vi "DAQ AI one shot ch 2 3.vi"(0 "device name":tag="Dev1", 1 "timeout (s)":dbl=1.0 format="%0.2f", 2 "stop (T)":bool=TRUE, 11 "error in":errorcluster, 12 "physical channels":string[](array[string])=["ai2", "ai3"], 13 "channel names":string[](array[string])=["Thermistor", "Heater"]) -> (4 "device name out":tag="Dev1", 6 "thermistor voltage":dbl, 10 "heater voltage":dbl, 14 "data":dynamicdata(waveform) caption="dynamic data", 15 "error out":errorcluster)   [LabVIEW 2019]
doc: "NI ELVIS \nAsynchronous AI one shot \nchannels 2 3 \nbug thermistor and heater\n\ncreated with DAQmx assistant\n\nPaul K Dixon\nP3600\nCSUSB Physics\n\n\nCreates, edits, and runs tasks using NI-DAQmx. Refer to the NI-DAQmx Readme for a complete listing of devices NI-DAQmx supports.\n\nWhen you place this Express VI on the block diagram, the DAQ Assistant launches to create a new task. After you create a task, you can double-click the DAQ Assistant Express VI to edit that task. For continuous measurement or generation, place a while loop around the DAQ Assistant Express VI."
uses:
  <vilib>/DAQmx/read.llb/DAQmx Read.vi
  <vilib>/DAQmx/read.llb/DAQmx Read (Analog 1D DBL NChan 1Samp).vi
  <vilib>/DAQmx/create/channels.llb/DAQmx Create Channel (TEDS-AI-Voltage-Basic).vi
  <vilib>/DAQmx/create/channels.llb/DAQmx Create Channel (AI-Voltage-Basic).vi
  <vilib>/DAQmx/miscellaneous.llb/DAQmx Fill In Error Info.vi
panel:
  # "DAQmx NI ELVIS \nAsynchronous AI one shot \nchannels 2 3  \nbug thermistor and heater"
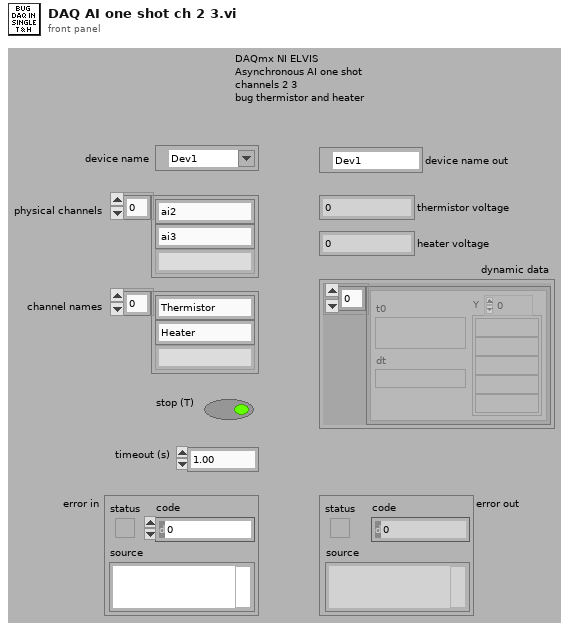
[diagram p1: front panel]
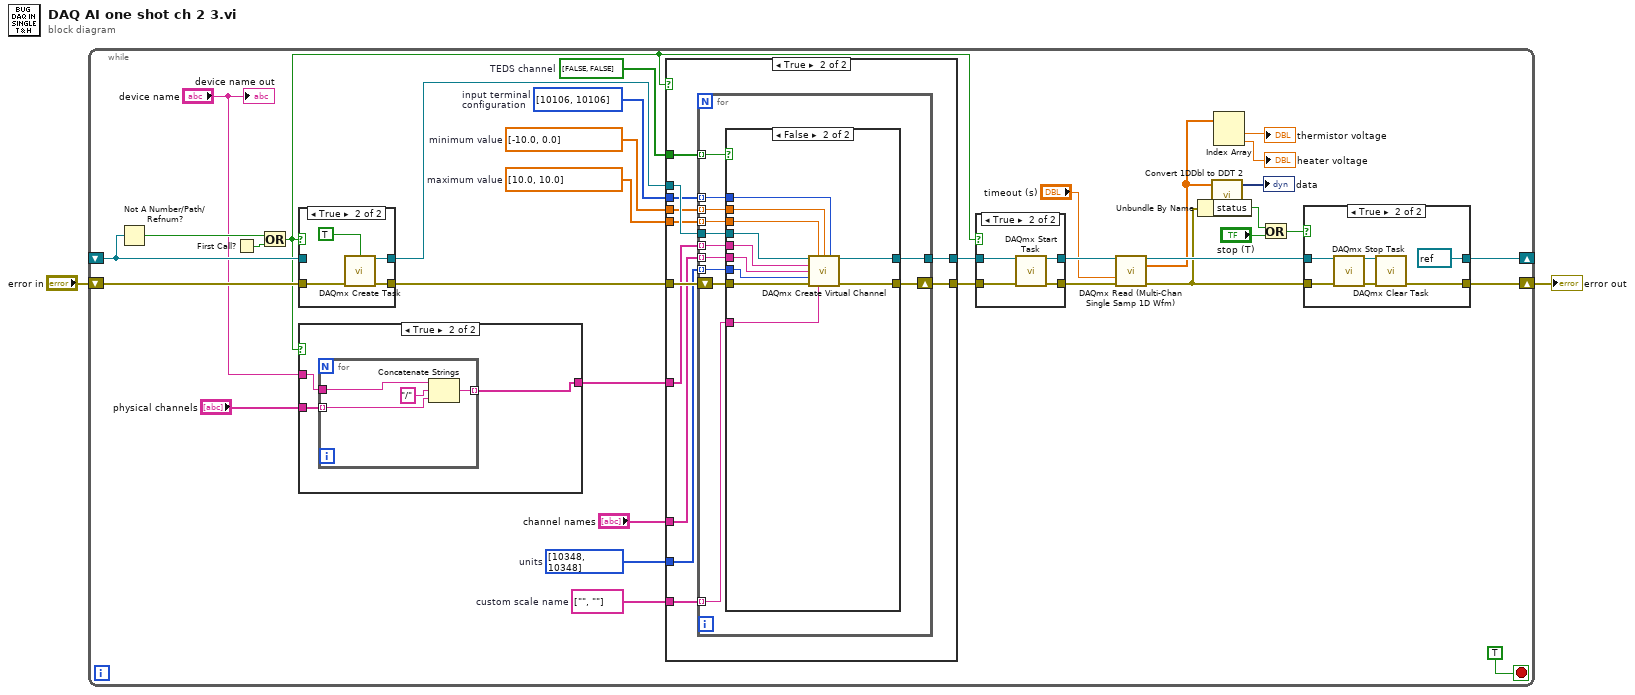
[diagram p0: block diagram]
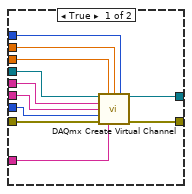
[diagram p5: hidden frame]
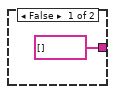
[diagram p6: hidden frame]
diagram:
  n1 = while {
    shift-right: [w12] -> _
    shift-left: _ -> [w33]
    shift-right: [w10] -> w1
    shift-left: "error in" -> [w34]
    stop <- TRUE stop-if-true
    w20 = bool[] [FALSE, FALSE]  # TEDS channel
    w21 = string[] ["", ""]  # custom scale name
    w22 = i32[] [10348, 10348] items=["Volts"=10348, "From TEDS"=12516, "From Custom Scale"=10065]  # units
    w25 = dbl[] [10.0, 10.0]  # maximum value
    w26 = dbl[] [-10.0, 0.0]  # minimum value
    w27 = i32[] [10106, 10106] items=["default"=-1, "RSE"=10083, "NRSE"=10078, "Differential"=10106, "Pseudodifferential"=12529]  # input terminal configuration
    n2 = Not A Number/Path/Refnum?(number/path/refnum=w33) -> (NaN/Path/Refnum?=w32:bool)
    n3 = First Call?() -> (First Call?: T/F=w35:bool)
    n4 = Or(x=w32, y=w35) -> (x .or. y?=w19:bool)
    n5 = case shown="True" w19 {
      tunnel: [w108 w112] -> w29
      tunnel: w33 -> [w108 _]
      tunnel: [w107 w111] -> w28
      tunnel: w34 -> [w107 w109]
      frame False {
      }
      frame True {
        n6 = call <vilib>:"DAQmx Create Task.vi"("auto cleanup"=TRUE, "error in"=w109) -> ("task out"=w112:refnum<k21>, "error out"=w111:errorcluster)  [unwired: 12 in]
      }
    }
    n7 = case shown="True" w19 {
      tunnel: [string[] [] w102] -> w24
      tunnel: "device name" -> [_ w101]
      tunnel: "physical channels" -> [_ w100]
      frame False {
      }
      frame True {
        n8 = for {
          tunnel: [w106] -> w102 mode=indexing
          tunnel: w101 -> [w105]
          tunnel: w100 -> [w103] mode=indexing
          n9 = Concatenate Strings(w105, "/" ("string"), w103) -> (w106:string)
        }
      }
    }
    n10 = case shown="True" w19 {
      tunnel: [w52 w62] -> w18
      tunnel: w29 -> [w52 w64]
      tunnel: [w51 w61] -> w17
      tunnel: w28 -> [w51 w63]
      tunnel: w27 -> [_ w60]
      tunnel: w26 -> [_ w59]
      tunnel: w25 -> [_ w58]
      tunnel: w24 -> [_ w57]
      tunnel: "channel names" -> [_ w56]
      tunnel: w22 -> [_ w55]
      tunnel: w21 -> [_ w54]
      tunnel: w20 -> [_ w53]
      frame False {
      }
      frame True {
        n11 = for {
          tunnel: w64 -> [w76]
          tunnel: [w74] -> w62
          tunnel: w60 -> [w72] mode=indexing
          tunnel: w59 -> [w71] mode=indexing
          tunnel: w58 -> [w70] mode=indexing
          tunnel: w57 -> [w69] mode=indexing
          tunnel: w56 -> [w68] mode=indexing
          tunnel: w55 -> [w67] mode=indexing
          tunnel: w54 -> [w66] mode=indexing
          shift-right: [w73] -> w61
          shift-left: w63 -> [w75]
          tunnel: w53 -> [w65] mode=indexing
          n12 = case shown="False" w65 {
            tunnel: w76 -> [w87 w98]
            tunnel: w75 -> [w86 w97]
            tunnel: [w85 w96] -> w74
            tunnel: [w84 w95] -> w73
            tunnel: w72 -> [w83 w94]
            tunnel: w71 -> [w82 w93]
            tunnel: w70 -> [w81 w92]
            tunnel: w69 -> [w80 w91]
            tunnel: w68 -> [w79 w90]
            tunnel: w67 -> [w78 w89]
            tunnel: w66 -> [w77 w88]
            frame True {
              n13 = call-poly <vilib>:"DAQmx Create Virtual Channel.vi"("task in"=w87, "maximum value"=w81, "minimum value"=w82, "input terminal configuration"=w83, "physical channels"=w80, "name to assign"=w79, "units"=w78, "error in"=w86, "custom scale name"=w77) -> ("task out"=w85:refnum<k21>, "error out"=w84:errorcluster)  [unwired: 5 in]
            }
            frame False {
              n14 = call-poly <vilib>:"DAQmx Create Virtual Channel.vi"("task in"=w98, "maximum value"=w92, "minimum value"=w93, "input terminal configuration"=w94, "physical channels"=w91, "name to assign"=w90, "units"=w89, "error in"=w97, "custom scale name"=w88) -> ("task out"=w96:refnum<k21>, "error out"=w95:errorcluster)  [unwired: 5 in]
            }
          }
        }
      }
    }
    n15 = case shown="True" w19 {
      tunnel: [w46 w49] -> w16
      tunnel: w18 -> [w46 w50]
      tunnel: [w45 w47] -> w15
      tunnel: w17 -> [w45 w48]
      frame False {
      }
      frame True {
        n16 = call <vilib>:"DAQmx Start Task.vi"("task/channels in"=w50, "error in"=w48) -> ("task out"=w49:refnum<k21>, "error out"=w47:errorcluster)  [unwired: 12 in]
      }
    }
    n17 = call-poly "DAQmx Read (Multi-Chan Single Samp 1D Wfm).vi"("task/channels in"=w16, "timeout"="timeout (s)", "error in"=w15) -> ("task out"=w11:refnum<k21>, "data"=w5:dbl[], "error out"=w9:errorcluster)  [unwired: 10 in]
    n18 = Unbundle By Name(w9) -> ("status"=w8:bool)
    n19 = call <vilib>:"Convert 1DDbl to DDT 2.vi"("Array"=w5) -> ("Dynamic Data Type"=→"data":dynamicdata)  [unwired: 3 in]
    n20 = Index Array(array=w5) -> (element #1=→"thermistor voltage":dbl, element #2=→"heater voltage":dbl)  [unwired: 2 in]
    n21 = Or(x=w8, y="stop (T)") -> (x .or. y?=w6:bool)
    n22 = case shown="True" w6 {
      tunnel: [w38 refnum<k21> refnum ("task in")] -> w12
      tunnel: w11 -> [w38 w44]
      tunnel: [w37 w41] -> w10
      tunnel: w9 -> [w37 w43]
      frame False {
      }
      frame True {
        n23 = call <vilib>:"DAQmx Stop Task.vi"("task/channels in"=w44, "error in"=w43) -> ("task out"=w40:refnum<k21>, "error out"=w42:errorcluster)  [unwired: 12 in]
        n24 = call <vilib>:"DAQmx Clear Task.vi"("task in"=w40, "error in"=w42) -> ("error out"=w41:errorcluster)  [unwired: 13 in]
      }
    }
    "device name out" <- "device name"
  }
  "error out" <- w1
